vi "Read Sweep Control.json.vi"(8 "error in (no error)":errorcluster, 10 "file (use dialog)":path, 11 "SweepControl in":refnum<class "SMO.SweepControl.lvclass">) -> (0 "error out":errorcluster, 2 "data":T1 {"Scan parameters"."Rate" format="%.2f"; "Scan parameters"."Step" format="%#_6p"; "Scan parameters"."End" format="%#_6p"; "Scan parameters"."Start" format="%#_6p"; "Repeat Experiment" min=1}, 3 "SweepControl out":refnum<class "SMO.SweepControl.lvclass">)   [LabVIEW 2019, in "SMO.SweepControl.lvclass"]
uses:
  SMO.SweepControl.lvclass
  <vilib>/addons/_JKI.lib/Serialization/JSON/JKI JSON Serialization.lvlib
  Typedefs/Enum - Action.ctl
  Typedefs/Enum - Priority.ctl
  Typedefs/Cluster - ScanControl.ctl
  Typedefs/ScanControl.ctl
  Typedefs/Cluster - ScanParamters.ctl
  Typedefs/ScanParamters.ctl
  Typedefs/Enum - Experiments.ctl
  Typedefs/Sweep Control JSON--Cluster.ctl
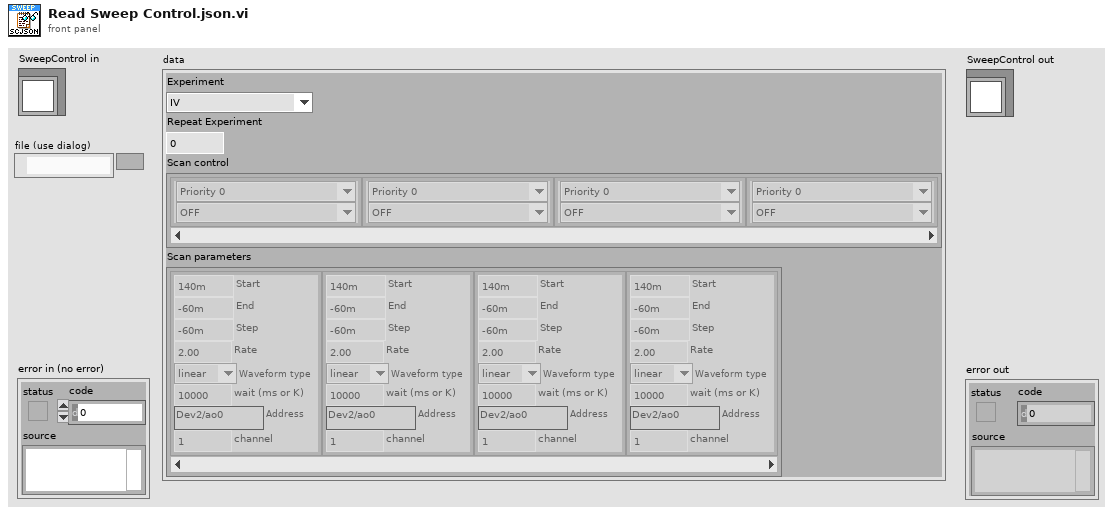
[diagram p1: front panel]
types:
  T1 = typedef "SMO.SweepControl.lvclass/Sweep Control JSON--Cluster.ctl" = cluster{"Experiment":T2, "Repeat Experiment":i32, "Scan control":T3, "Scan parameters":T7}
  T2 = typedef "SMO.SweepControl.lvclass/Enum - Experiments.ctl" = enum16{"IV", "IV_Fast", "THz_DelayLine", "Lockin_Vsg", "Lockin_Sweep", "Lockin_Time", "AI WFM time", "Lockin (experimental)"}
  T3 = typedef "SMO.SweepControl.lvclass/ScanControl.ctl" = T4[]
  T4 = typedef "SMO.SweepControl.lvclass/Cluster - ScanControl.ctl" = cluster{"Priority":T5, "Scan name":T6}
  T5 = typedef "SMO.SweepControl.lvclass/Enum - Priority.ctl" = enum16{"Priority 0", "Priority 1", "Priority 2", "Priority 3", "Priority 4", "Priority 5"}
  T6 = typedef "SMO.SweepControl.lvclass/Enum - Action.ctl" = enum16{"OFF", "time", "Lockin Amplitude", "Lockin Frequency", "Lockin Bias", "Delay", "Strain", "DAQ Bias", "Magnet Field", "Temperature", "MW f1", "MW f2", "MW Amplitude1", "MW Amplitude2"}
  T7 = typedef "SMO.SweepControl.lvclass/ScanParamters.ctl" = T8[]
  T8 = typedef "SMO.SweepControl.lvclass/Cluster - ScanParamters.ctl" = cluster{"Start":dbl, "End":dbl, "Step":dbl, "Rate":dbl, "Waveform type":enum16{"linear", "triangle", "power"}, "wait (ms or K)":dbl, "Address":string, "channel":i32}
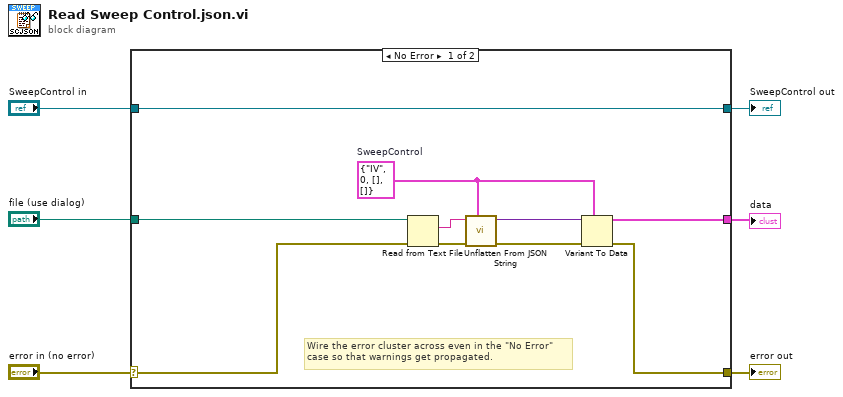
[diagram p0: block diagram]
diagram:
  n1 = case shown="No Error" "error in (no error)" {
    selector: "error in (no error)" -> [w13 w18]
    tunnel: [w11 w18] -> w5
    tunnel: [w16 w17] -> w3
    tunnel: "SweepControl in" -> [w16 w17]
    tunnel: "file (use dialog)" -> [w8 _]
    tunnel: [w7 _] -> w1
    frame No Error {
      w9 = T1 {"Experiment"=enum."IV", "Repeat Experiment"=0, "Scan control"=[], "Scan parameters"=[]}  # SweepControl
      # "Wire the error cluster across even in the \"No Error\"\ncase so that warnings get propagated."
      n2 = Read from Text File(file (use dialog)=w8, error in=w13) -> (text=w14:string, error out=w15:errorcluster)  [unwired: 2 in, 2 out]
      n3 = call <vilib>:"Unflatten From JSON String.vi"("Type and Defaults"=w9, "error in (no error)"=w15, "JSON String"=w14) -> ("error out"=w12:errorcluster, "Variant"=w10:variant)  [unwired: 7 in]
      n4 = Variant To Data(error in=w12, type=w9, Variant=w10) -> (data=w7:T1, error out=w11:errorcluster)
    }
    frame Error {
    }
  }
  "error out" <- w5
  "SweepControl out" <- w3
  "data" <- w1
